vi "CRYInsert Value.vi"(8 "sOptionUpdate":string, 9 "sOption":string, 10 "Index":i32[](array[numeric]), 11 "Value":T1 {"Z data" items=["dB", "Lin"]; "X data" items=["dB", "Lin"]; "Y data" items=["dB", "Lin"]; "Z dB ref" format="%.1f"; "Z axis" items=["Log", "Lin"]; "X dB ref" format="%.1f"; "X axis" items=["Log", "Lin"]; "Y axis" items=["Log", "Lin"]; "Y dB ref" format="%.1f"; "Curve"."z" format="%.2f"; "Curve"."y" format="%.2f"; "Curve"."x" format="%.2f"}) -> (2 "Inserted Index":i32[](array[numeric]), 3 "Inserted Name Out":string[](array[string]))   [LabVIEW 2013]
uses:
  CRYSystem/Typedef Control/CRYData Cluster Array.ctl
  CRYSystem/Typedef Control/CRYData Cluster.ctl
  Global/CRYCurve Library Global.vi
  Global/CRYCurves Array Global.vi
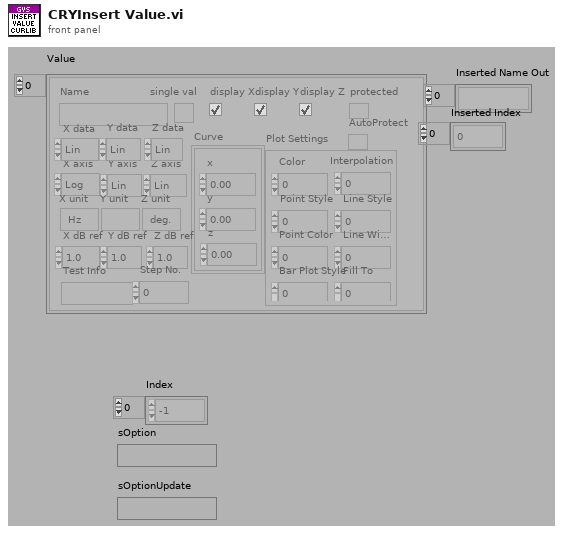
[diagram p1: front panel]
types:
  T1 = typedef "CRYData Cluster Array.ctl" = T2[]
  T2 = typedef "CRYData Cluster.ctl" = cluster{"Name":string, "Curve":cluster{"x":dbl, "y":dbl, "z":dbl}[], "X data":u16, "Y data":u16, "Z data":u16, "X axis":u16, "Y axis":u16, "Z axis":u16, "X unit":string, "Y unit":string, "Z unit":string, "X dB ref":dbl, "Y dB ref":dbl, "Z dB ref":dbl, "single val":bool, "protected":bool, "display X":bool, "display Y":bool, "display Z":bool, "Test Info":string, "Step No.":i32, "Plot Settings":cluster{"Color":u32, "Interpolation":u8, "Point Style":u8, "Line Style":u8, "Point Color":u32, "Line Width":u8, "Bar Plot Style":u8, "Fill To":i16}, "AutoProtect":bool}
  T3 = cluster{"CurveOld":string[], "ValueOld":string[], "ResultOld":string[], "WFMOld":string[], "CurveNew":string[], "ValueNew":string[], "ResultNew":string[], "WFMNew":string[]}
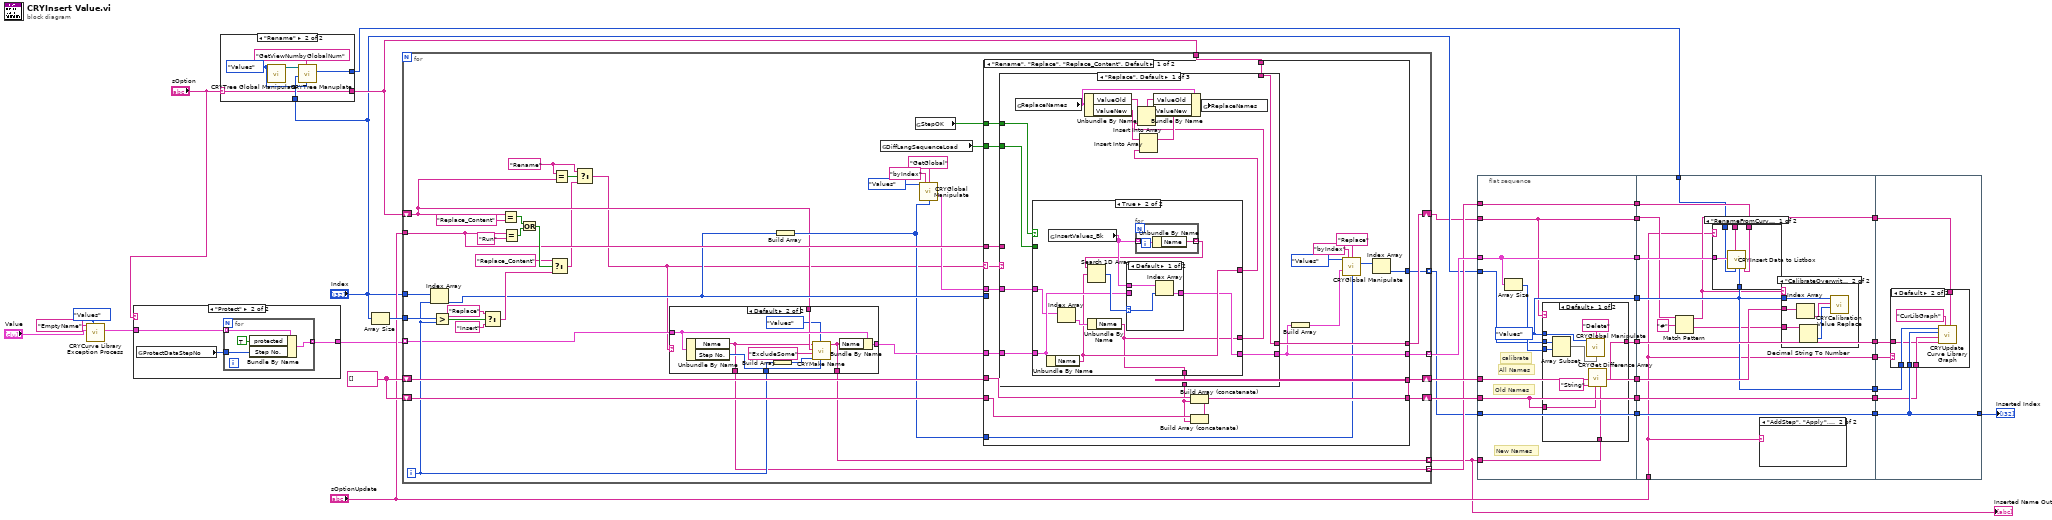
[diagram p0: block diagram]
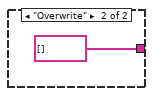
[diagram p4: hidden frame]
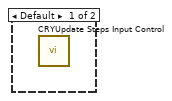
[diagram p5: hidden frame]
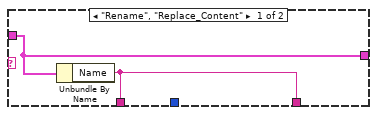
[diagram p9: hidden frame]
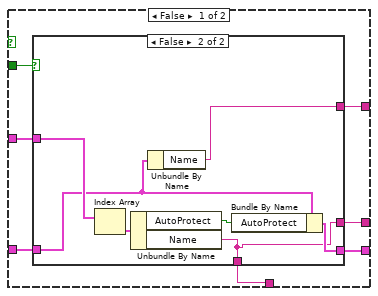
[diagram p10: hidden frame]
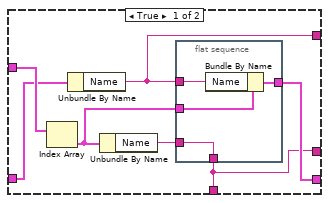
[diagram p11: hidden frame]
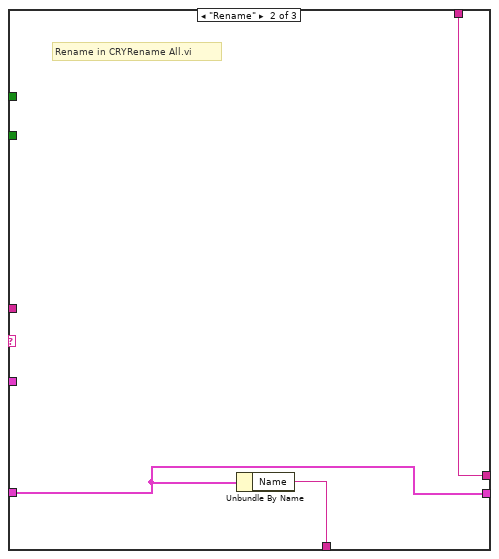
[diagram p13: hidden frame]
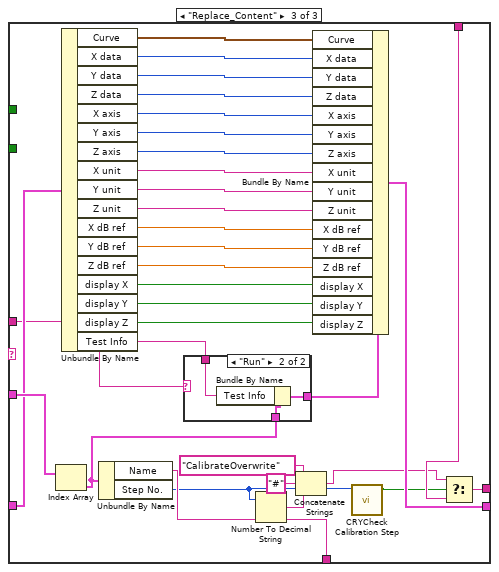
[diagram p14: hidden frame]
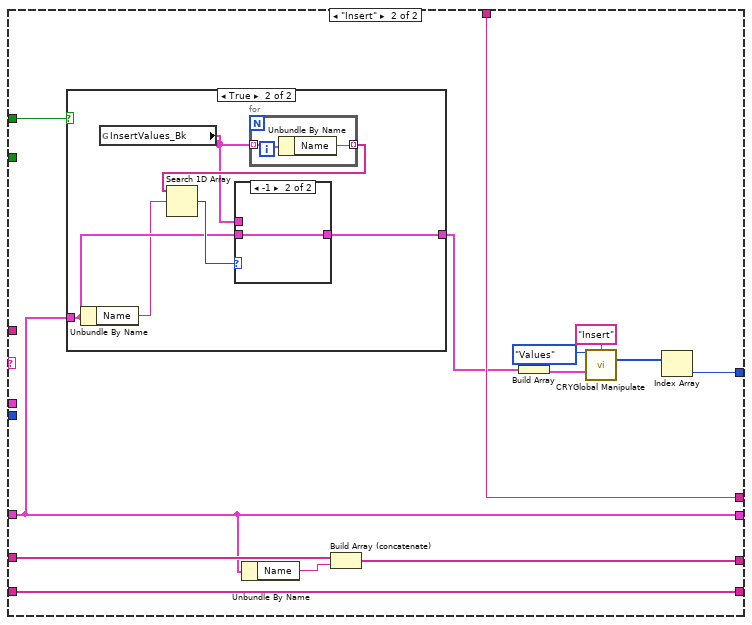
[diagram p16: hidden frame]
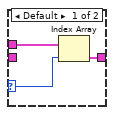
[diagram p18: hidden frame]
diagram:
  w25 = string[] []
  n1 = call "CRYCurve Library Exception Process.vi"("Type In"=enum16{"Curves", "Values", "Results", "WFM"}."Values", "Curve/Value"="Value", "sAction"="EmptyName") -> ("Curve/Value Out"=w1:T1)  [unwired: 6 in, 2 out]
  n2 = case shown="\"Protect\"" "sOption" {
    tunnel: w1 -> [w35 w38]
    tunnel: [w35 w37] -> w8
    frame Default {
    }
    frame "Protect" {
      n3 = global read "CRYCurve Library Global.vi" "ProtectDataStepNo"() -> (w36:i32)
      n4 = for {
        tunnel: w38 -> [w42] mode=indexing
        tunnel: [w41] -> w37 mode=indexing
        tunnel: w36 -> [w39]
        n5 = Bundle By Name(cluster=w42, "protected"=TRUE, "Step No."=w39) -> (w41:T2)
      }
    }
  }
  n6 = case shown="\"Rename\"" "sOption" {
    selector: "sOption" -> [w43 w45]
    tunnel: "Index" -> [_ w46]
    tunnel: [_ w47] -> w11
    tunnel: [w43 w45] -> w12
    frame Default {
    }
    frame "Rename" {
      w44 = enum16{"Curves", "Values", "Results", "WFM"}."Values" ("Type In")
      n7 = call "CRYTree Global Manipulate.vi"("Type In"=w44) -> ("Tree/Curve Tree"=w48:refnum<vi>)  [unwired: 7 in, 3 out]
      n8 = call "CRYTree Manuplate.vi"("Type"=w44, "sAction"="GetViewNumbyGlobalNum", "nData"=w46, "Tree in"=w48) -> ("nData Out"=w47:i32[])  [unwired: 4 in, 3 out]
    }
  }
  n9 = Array Size(array="Index") -> (size(s)=w19:i32)
  n10 = for {
    tunnel: [w77] -> w5 mode=indexing
    tunnel: "Index" -> [w76]
    tunnel: w8 -> [w66] mode=indexing
    tunnel: [w82] -> w33 mode=indexing
    tunnel: w19 -> [w87]
    shift-right: [w85] -> w32
    shift-left: w25 -> [w86]
    shift-right: [w83] -> w21
    shift-left: w25 -> [w84]
    tunnel: w12 -> [w75]
    tunnel: "sOptionUpdate" -> [w67]
    tunnel: [w59] -> w14 mode=indexing
    shift-right: [w53] -> w9
    shift-left: w12 -> [w56]
    tunnel: [w51] -> w6 mode=indexing
    i -> [w74]
    w58 = "Rename" ("y")
    n11 = Index Array(array=w76, index=w74) -> (element=w65:i32)
    n12 = Greater?(x=w87, y=w74) -> (0:w79:bool)
    n13 = Select(t="Replace" ("sOption"), s=w79, f="Insert" ("sOption")) -> (s? t:f=w78:string)
    n14 = Equal?(x=w56, y="Replace_Content") -> (x = y?=w71:bool)
    n15 = Equal?(x=w67, y="Run") -> (x = y?=w70:bool)
    n16 = Or(x=w71, y=w70) -> (x .or. y?=w69:bool)
    n17 = Select(t="Replace_Content" ("y"), s=w69, f=w78) -> (s? t:f=w55:string)
    n18 = Equal?(x=w58, y=w56) -> (x = y?=w57:bool)
    n19 = Select(t=w58, s=w57, f=w55) -> (s? t:f=w54:string)
    n20 = case shown="Default" w54 {
      tunnel: [w90 w100] -> w88
      tunnel: w66 -> [w90 w99]
      tunnel: [w89 w98] -> w77
      tunnel: w56 -> [_ w97]
      tunnel: w74 -> [_ w92]
      tunnel: [w89 w91] -> w59
      frame "Rename", "Replace_Content" {
        n21 = Unbundle By Name(w90) -> ("Name"=w89:string)
      }
      frame Default {
        n22 = Unbundle By Name(w99) -> ("Name"=w91:string, "Step No."=w93:i32)
        n23 = Build Array(w92) -> (w95:i32[])
        n24 = call "CRYMake Name.vi"("Step No."=w93, "Type"=enum16{"Curves", "Values", "Results", "WFM"}."Values", "nData"=w95, "sOption"="ExcludeSome", "sAction"=w97, "Name In"=w91) -> ("Name Out"=w98:string)  [unwired: 4 in, 1 out]
        n25 = Bundle By Name(cluster=w99, "Name"=w98) -> (w100:T2)
      }
    }
    n26 = Build Array(w65) -> (w61:i32[])
    n27 = global read "CRYCurve Library Global.vi" "DiffLangSequenceLoad"() -> (w52:bool)
    n28 = global read "CRYCurve Library Global.vi" "StepOK"() -> (w50:bool)
    n29 = call "CRYGlobal Manipulate.vi"("Type"=enum16{"Curves", "Values", "Results", "WFM"}."Values", "sOption"="byIndex", "sAction"="GetGlobal", "nData"=w61) -> ("Values Out"=w64:T2[])  [unwired: 5 in, 6 out]
    n30 = case shown="\"Rename\", \"Replace\", \"Replace_Content\", Default" w54 {
      selector: w54 -> [w112 _]
      tunnel: w64 -> [w120 _]
      tunnel: w88 -> [w121 w217]
      tunnel: w65 -> [_ _]
      tunnel: [w118 w228] -> w85
      tunnel: w86 -> [w119 w228]
      tunnel: w84 -> [w117 w227]
      tunnel: [w115 w226] -> w83
      tunnel: [w108 w217] -> w82
      tunnel: [w114 w224] -> w53
      tunnel: w75 -> [w113 w224]
      tunnel: w67 -> [w111 _]
      tunnel: w61 -> [w107 _]
      tunnel: w52 -> [w104 _]
      tunnel: [w102 w219] -> w51
      tunnel: w50 -> [w101 w218]
      frame "Rename", "Replace", "Replace_Content", Default {
        n31 = case shown="\"Replace\", Default" w112 {
          tunnel: w121 -> [w134 w177 w209]
          tunnel: w120 -> [w136 _ w211]
          tunnel: [w135 w179 w195] -> w116
          tunnel: [w133 w177 w210] -> w108
          tunnel: [w132 w178 w198] -> w114
          tunnel: w113 -> [w132 w178 w197]
          tunnel: w111 -> [_ _ w186]
          tunnel: w104 -> [w131 _ _]
          tunnel: w101 -> [w122 _ _]
          frame "Replace", Default {
            n32 = global read "CRYCurve Library Global.vi" "ReplaceNames"() -> (w130:T3)
            n33 = case shown="True" w122 {
              tunnel: w136 -> [w143 w165]
              tunnel: [w142 w162] -> w135
              tunnel: w134 -> [w141 w166]
              tunnel: [w140 w163] -> w133
              tunnel: w131 -> [w139 _]
              tunnel: [w138 w164] -> w124
              tunnel: [w137 w162] -> w123
              frame False {
                n34 = case shown="False" w139 {
                  tunnel: w143 -> [w150 w161]
                  tunnel: [w145 w155] -> w142
                  tunnel: w141 -> [w148 w157]
                  tunnel: [w149 w158] -> w140
                  tunnel: [w145 w155] -> w137
                  tunnel: [w144 w156] -> w138
                  frame True {
                    n35 = Index Array(array=w150) -> (element=w147:T2)  [unwired: 1 in]
                    n36 = Unbundle By Name(w148) -> ("Name"=w144:string)
                    n37 = Unbundle By Name(w147) -> ("Name"=w146:string)
                    n38 = flat-sequence {
                      tunnel: [w154] -> w149
                      tunnel: w147 -> [w153]
                      tunnel: w144 -> [w152]
                      tunnel: [w151] -> w145
                      tunnel: w146 -> [w151]
                      frame #0 {
                        n39 = Bundle By Name(cluster=w153, "Name"=w152) -> (w154:T2)
                      }
                    }
                  }
                  frame False {
                    n40 = Index Array(array=w161) -> (element=w160:T2)  [unwired: 1 in]
                    n41 = Unbundle By Name(w160) -> ("AutoProtect"=w159:bool, "Name"=w155:string)
                    n42 = Unbundle By Name(w157) -> ("Name"=w156:string)
                    n43 = Bundle By Name(cluster=w157, "AutoProtect"=w159) -> (w158:T2)
                  }
                }
              }
              frame True {
                n44 = Unbundle By Name(w166) -> ("Name"=w164:string)
                n45 = global read "CRYCurves Array Global.vi" "InsertValues_Bk"() -> (w169:T1)
                n46 = Index Array(array=w165) -> (element=w170:T2)  [unwired: 1 in]
                n47 = Unbundle By Name(w170) -> ("Name"=w162:string)
                n48 = for {
                  tunnel: w169 -> [w176] mode=indexing
                  tunnel: [w175] -> w167 mode=indexing
                  n49 = Unbundle By Name(w176) -> ("Name"=w175:string)
                }
                n50 = Search 1D Array(1D array=w167, element=w164) -> (index of element=w168:i32)  [unwired: 1 in]
                n51 = case shown="Default" w168 {
                  selector: w168 -> [w172 _]
                  tunnel: w169 -> [w173 _]
                  tunnel: [w171 w174] -> w163
                  tunnel: w166 -> [_ w174]
                  frame Default {
                    n52 = Index Array(array=w173, index=w172) -> (element=w171:T2)
                  }
                  frame -1 {
                  }
                }
              }
            }
            n53 = Unbundle By Name(w130) -> ("ValueOld"=w128:string[], "ValueNew"=w127:string[])
            n54 = Insert Into Array(array=w128, new element=w123) -> (w126:string[])  [unwired: 1 in]
            n55 = Insert Into Array(array=w127, new element=w124) -> (w125:string[])  [unwired: 1 in]
            n56 = Bundle By Name(cluster=w130, "ValueOld"=w126, "ValueNew"=w125) -> (w129:T3)
            n57 = global write "CRYCurve Library Global.vi" "ReplaceNames"(w129) -> ()
          }
          frame "Rename" {
            # "Rename in CRYRename All.vi"
            n58 = Unbundle By Name(w177) -> ("Name"=w179:string)
          }
          frame "Replace_Content" {
            n59 = Index Array(array=w211) -> (element=w185:T2)  [unwired: 1 in]
            n60 = Unbundle By Name(w209) -> ("Curve"=w208:cluster{"x":dbl, "y":dbl, "z":dbl}[], "X data"=w207:u16, "Y data"=w206:u16, "Z data"=w205:u16, "X axis"=w204:u16, "Y axis"=w203:u16, "Z axis"=w202:u16, "X unit"=w201:string, "Y unit"=w200:string, "Z unit"=w199:string, "X dB ref"=w189:dbl, "Y dB ref"=w188:dbl, "Z dB ref"=w187:dbl, "display X"=w182:bool, "display Y"=w181:bool, "display Z"=w180:bool, "Test Info"=w183:string)
            n61 = Unbundle By Name(w185) -> ("Name"=w195:string, "Step No."=w191:i32)
            n62 = case shown="\"Run\"" w186 {
              tunnel: w185 -> [w212 w215]
              tunnel: [w212 w214] -> w184
              tunnel: w183 -> [_ w213]
              frame Default {
              }
              frame "Run" {
                n63 = Bundle By Name(cluster=w215, "Test Info"=w213) -> (w214:T2)
              }
            }
            n64 = Number To Decimal String(number=w191) -> (decimal integer string=w192:string)  [unwired: 1 in]
            n65 = Concatenate Strings("CalibrateOverwrite" ("f"), "#" ("string"), w192) -> (w190:string)
            n66 = Bundle By Name(cluster=w184, "Curve"=w208, "X data"=w207, "Y data"=w206, "Z data"=w205, "X axis"=w204, "Y axis"=w203, "Z axis"=w202, "X unit"=w201, "Y unit"=w200, "Z unit"=w199, "X dB ref"=w189, "Y dB ref"=w188, "Z dB ref"=w187, "display X"=w182, "display Y"=w181, "display Z"=w180) -> (w210:T2)
            n67 = call "CRYCheck Calibration Step.vi"("Step No"=w191) -> ("Is Calibration?"=w196:bool)  [unwired: 9 in, 1 out]
            n68 = Select(t=w190, s=w196, f=w197) -> (s? t:f=w198:string)
          }
        }
        n69 = Build Array (concatenate)(w119, w116) -> (w118:string[])
        n70 = Build Array (concatenate)(w117, w116) -> (w115:string[])
        n71 = Build Array(w108) -> (w105:T2[])
        n72 = call "CRYGlobal Manipulate.vi"("Type"=enum16{"Curves", "Values", "Results", "WFM"}."Values", "sOption"="byIndex", "sAction"="Replace", "Values"=w105, "nData"=w107) -> ("nData out"=w103:i32[])  [unwired: 4 in, 6 out]
        n73 = Index Array(array=w103) -> (element=w102:i32)  [unwired: 1 in]
      }
      frame "Insert" {
        n74 = case shown="True" w218 {
          tunnel: w217 -> [w229 w232]
          tunnel: [w229 w231] -> w216
          frame False {
          }
          frame True {
            n75 = Unbundle By Name(w232) -> ("Name"=w230:string)
            n76 = global read "CRYCurves Array Global.vi" "InsertValues_Bk"() -> (w233:T1)
            n77 = for {
              tunnel: w233 -> [w241] mode=indexing
              tunnel: [w240] -> w235 mode=indexing
              n78 = Unbundle By Name(w241) -> ("Name"=w240:string)
            }
            n79 = Search 1D Array(1D array=w235, element=w230) -> (index of element=w234:i32)  [unwired: 1 in]
            n80 = case shown="-1" w234 {
              selector: w234 -> [w237 _]
              tunnel: w233 -> [w238 _]
              tunnel: [w236 w239] -> w231
              tunnel: w232 -> [_ w239]
              frame Default {
                n81 = Index Array(array=w238, index=w237) -> (element=w236:T2)
              }
              frame -1 {
              }
            }
          }
        }
        n82 = Unbundle By Name(w217) -> ("Name"=w225:string)
        n83 = Build Array (concatenate)(w227, w225) -> (w226:string[])
        n84 = Build Array(w216) -> (w221:T2[])
        n85 = call "CRYGlobal Manipulate.vi"("Type"=enum16{"Curves", "Values", "Results", "WFM"}."Values", "sAction"="Insert", "Values"=w221) -> ("nData out"=w220:i32[])  [unwired: 6 in, 6 out]
        n86 = Index Array(array=w220) -> (element=w219:i32)  [unwired: 1 in]
      }
    }
  }
  "Inserted Name Out" <- w5
  n87 = flat-sequence {
    tunnel: [w252] -> w34
    tunnel: w33 -> [w252]
    tunnel: "Index" -> [w249]
    tunnel: w32 -> [w242]
    tunnel: [w251] -> w31
    tunnel: [w242] -> w30
    tunnel: [w248] -> w27
    tunnel: [w244] -> w24
    tunnel: [w247] -> w22
    tunnel: w21 -> [w247]
    tunnel: [w245] -> w20
    tunnel: [w246] -> w15
    tunnel: w14 -> [w246]
    tunnel: w9 -> [w245]
    tunnel: w6 -> [w244]
    tunnel: w5 -> [w243]
    tunnel: [w275] -> w29
    tunnel: [w274] -> w28
    tunnel: w30 -> [w274]
    tunnel: w31 -> [w275]
    tunnel: w34 -> [w273]
    tunnel: w27 -> [w270]
    tunnel: [w270] -> w26
    tunnel: w24 -> [w272]
    tunnel: [w272] -> w23
    tunnel: w22 -> [w271]
    tunnel: w20 -> [w266]
    tunnel: [w263] -> w17
    tunnel: "sOptionUpdate" -> [w263]
    tunnel: w15 -> [w267]
    tunnel: [w264] -> w13
    tunnel: w11 -> [w265]
    tunnel: w29 -> [w288]
    tunnel: w28 -> [w289]
    tunnel: w26 -> [w291]
    tunnel: w23 -> [w290]
    tunnel: [w290] -> w18
    tunnel: w17 -> [w287]
    tunnel: w13 -> [w286]
    frame #0 {
      w248 = enum16{"Curves", "Values", "Results", "WFM"}."Values" ("Type")
      # "New Names"
      # "Old Names"
      # "All Names"
      # "calibrate"
      n88 = Array Size(array=w252) -> (size(s)=w250:i32)
      n89 = case shown="Default" w245 {
        tunnel: [w253 string[] [] ("Deleted Names")] -> w251
        tunnel: w250 -> [w261 _]
        tunnel: w249 -> [w260 _]
        tunnel: w248 -> [w257 _]
        tunnel: w243 -> [w255 _]
        tunnel: w242 -> [w254 _]
        frame Default {
          n90 = Array Subset(array=w260, index=w261) -> (w258:i32[])  [unwired: 1 in]
          n91 = call "CRYGlobal Manipulate.vi"("Type"=w257, "sAction"="Delete", "nData"=w258) -> ()  [unwired: 6 in, 7 out]
          n92 = call "CRYGet Difference Array.vi"("String2"=w255, "String1"=w254, "sOption"="String") -> ("StringDiff Out"=w253:string[])  [unwired: 7 in, 1 out]
        }
        frame "Overwrite" {
        }
      }
    }
    frame #1 {
      n93 = Match Pattern(string=w266, regular expression="#" ("string")) -> (before substring=w264:string, after substring=w268:string)  [unwired: 1 in, 2 out]
      n94 = case shown="\"RenameFromCurve\", Default" w263 {
        tunnel: w273 -> [w280 _]
        tunnel: w270 -> [w279 _]
        tunnel: w267 -> [w278 _]
        tunnel: w264 -> [w277 _]
        tunnel: w265 -> [w276 _]
        frame "RenameFromCurve", Default {
          n95 = call "CRYInsert Data to Listbox.vi"("OrgNames"=w278, "Type"=w279, "nData"=w276, "sOption"=w277, "Values"=w280) -> ()  [unwired: 6 in, 1 out]
        }
        frame "Run" {
        }
      }
      n96 = case shown="\"AddStep\", \"Apply\", \"Run\"" w263 {
        frame Default {
          n97 = call "CRYUpdate Steps Input Control.vi"() -> ()  [unwired: 12 in]
        }
        frame "AddStep", "Apply", "Run" {
        }
      }
      n98 = case shown="\"CalibrateOverwrite\"" w264 {
        tunnel: w271 -> [_ w284]
        tunnel: w270 -> [_ w283]
        tunnel: w268 -> [_ w282]
        frame Default {
        }
        frame "CalibrateOverwrite" {
          n99 = Index Array(array=w284) -> (element=w285:string)  [unwired: 1 in]
          n100 = Decimal String To Number(string=w282) -> (number=w281:i32)  [unwired: 2 in, 1 out]
          n101 = call "CRYCalibration Value Replace.vi"("Step No."=w281, "Corr/EQ/Sens Name"=w285, "Type"=w283) -> ()  [unwired: 9 in]
        }
      }
    }
    frame #2 {
      n102 = case shown="Default" w287 {
        tunnel: w291 -> [_ w296]
        tunnel: w290 -> [_ w295]
        tunnel: w289 -> [_ w294]
        tunnel: w288 -> [_ w293]
        tunnel: w286 -> [_ w292]
        frame "RenameFromCurve", "Run" {
        }
        frame Default {
          n103 = call "CRYUpdate Curve Library Graph.vi"("sOption 2"=w292, "sOption 1"="CurLibGraph" ("sOption"), "Deleted Names"=w293, "Replaced Old Names"=w294, "Index"=w295, "Type"=w296) -> ()  [unwired: 6 in]
        }
      }
    }
  }
  "Inserted Index" <- w18
